vi "MQTT_PingResp.vi"(8 "error in (no error)":errorcluster) -> (0 "error out":errorcluster, 2 "PingResp Message":u8[](array[numeric]) format="%x")   [LabVIEW 2018, in "AWS_IoT.lvlib"]
doc: "This VI responds to a PINREQ message and corresponds to a \"PING\" reply. \n\n© 2015 - daq.io, LLC - Peter Adelhardt"
uses:
  AWS_IoT.lvlib
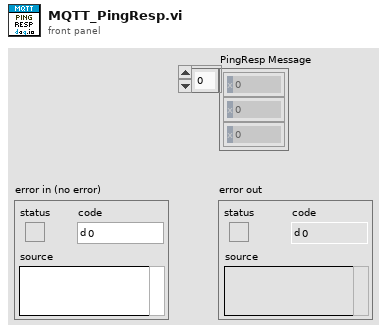
[diagram p1: front panel]
types:
  T1 = typedef "AWS_IoT.lvlib/Retain_Flag.ctl" = bool
  T2 = typedef "AWS_IoT.lvlib/QoS.ctl" = enum8{"At most once", "At least once", "Exactly once", "Reserved"}
  T3 = typedef "AWS_IoT.lvlib/DUP_Flag.ctl" = bool
  T4 = typedef "AWS_IoT.lvlib/MessageType.ctl" = enum32{"Reserved", "CONNECT", "CONNACK", "PUBLISH", "PUBACK", "PUBREC", "PUBREL", "PUBCOMP", "SUBSCRIBE", "SUBACK", "UNSUBSCRIBE", "UNSUBACK", "PINGREQ", "PINGRESP", "DISCONNECT", "Reserved2"}
  T5 = typedef "AWS_IoT.lvlib/SSL_Connection.ctl" = cluster{"connection ID":refnum<k5>, "TLS":cluster{"CXT ptr":i32, "SSL ptr":i32, "Socket ptr":i32}, "NIssleay library path":path, "server url":string}
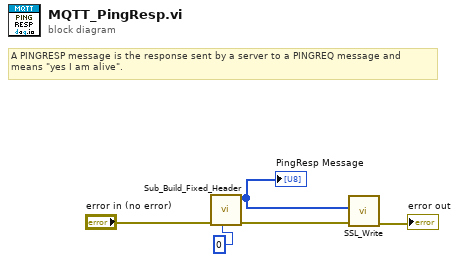
[diagram p0: block diagram]
diagram:
  # "A PINGRESP message is the response sent by a server to a PINGREQ message and\nmeans \"yes I am alive\"."
  n1 = call "Sub_Build_Fixed_Header.vi"("Remaining Length"=u32 0, "error in (no error)"="error in (no error)") -> ("error out"=w5:errorcluster, "Fixed Header"=w1:u8[], "Retain"=w10:T1, "QoS"=w9:T2, "DUP"=w8:T3, "MessageType"=w11:T4)  [unwired: 4 in]
  "PingResp Message" <- w1
  n2 = call "SSL_Write.vi"("error in (no error)"=w5, "data in"=w1) -> ("error out"=→"error out":errorcluster, "SSL_Connection"=w2:T5, 7:w3)  [unwired: 7 in]
